vi "initialize.vi"(7 "mode":T1, 8 "log path":path, 9 "pathCtrl":path=path "/Users/philippe/Desktop/LV_Quanser/biquadsff.so", 10 "pathDataCtrl":path=path "/Users/philippe/Desktop/LV_Quanser/biquadsff.so") -> (3 "Qube":refnum<class "Qube.lvclass">)   [LabVIEW 2020, in "Qube.lvclass"]
uses:
  Qube.lvclass
  mode.ctl
  Qube.lvclass/Qube.ctl
  <vilib>/Quanser/Rapid Control Prototyping Toolkit/hardware/HIL Board/HIL Board.lvclass
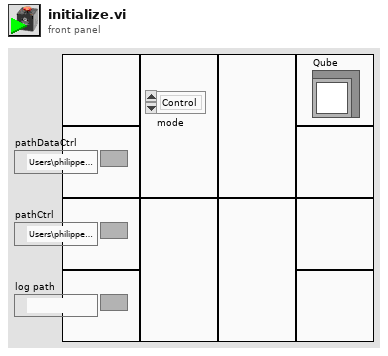
[diagram p1: front panel]
types:
  T1 = typedef "Qube.lvclass/mode.ctl" = enum16{"Control", "Identify"}
  T2 = enum16{"open", "replace", "create", "open or create", "replace or create", "replace or create with confirmation"}
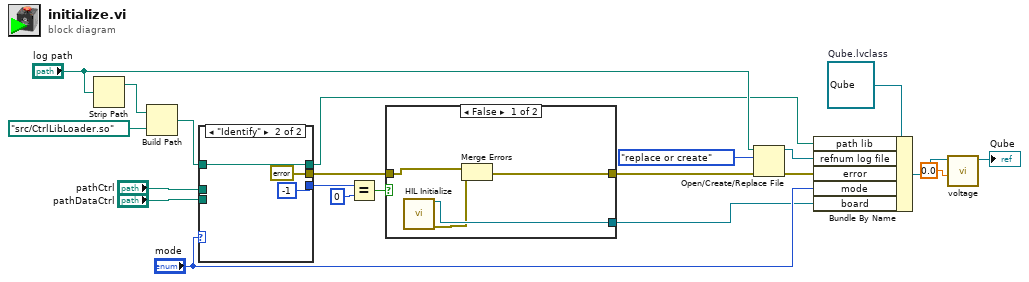
[diagram p0: block diagram]
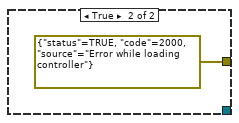
[diagram p2: hidden frame]
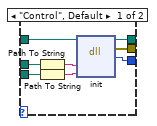
[diagram p3: hidden frame]
diagram:
  w20 = refnum<class "Qube.lvclass"> refnum  # Qube.lvclass
  n1 = Strip Path(path="log path") -> (stripped path=w16:path)  [unwired: 1 out]
  n2 = Build Path(base path=w16, name or relative path=path "src/CtrlLibLoader.so") -> (appended path=w13:path)
  n3 = case shown="\"Identify\"" "mode" {
    tunnel: "pathCtrl" -> [w26 _]
    tunnel: [w23 w31] -> w2
    tunnel: [w24 errorcluster {"status"=FALSE, "code"=0, "source"=""} ("error out")] -> w4
    tunnel: "pathDataCtrl" -> [w27 _]
    tunnel: w13 -> [w25 w31]
    tunnel: [w22 -1 ("return type")] -> w7
    frame "Control", Default {
      n4 = Path To String(path=w26) -> (string=w28:string)
      n5 = Path To String(path=w27) -> (string=w29:string)
      n6 = dll-call lib="Users/philippe/Desktop/cpp/LibLoader/libLoader.so" fn="init"(path in=w25, "pathLib"=w28, "pathInit"=w29) -> (path out=w23:path, error out=w24:errorcluster, "return type"=w22:i32)  [unwired: 4 in]
    }
    frame "Identify" {
    }
  }
  n7 = Equal?(x=w7, y=0) -> (x = y?=w5:bool)
  n8 = case shown="False" w5 {
    tunnel: w4 -> [w34 _]
    tunnel: [w35 errorcluster {"status"=TRUE, "code"=2000, "source"="Error while loading controller"} ("error out")] -> w3
    tunnel: [w36 _] -> w1
    frame False {
      n9 = call "HIL Initialize"() -> ("board out"=w36:refnum<class "HIL Board.lvclass">, "error out"=w33:errorcluster)  [unwired: 14 in]
      n10 = Merge Errors(w34, w33) -> (w35:errorcluster)
    }
    frame True {
    }
  }
  n11 = Open/Create/Replace File(file path (use dialog)="log path", error in=w3, operation (0:open)=T2."replace or create") -> (refnum out=w11:refnum<file>, error out=w10:errorcluster)  [unwired: 3 in, 1 out]
  n12 = Bundle By Name(cluster=w20, "path lib"=w2, "refnum log file"=w11, "error"=w10, "mode"="mode", "board"=w1) -> (w19:refnum<class "Qube.lvclass">)
  n13 = call "voltage.vi"("u"=0.0, "Qube"=w19) -> ("Qube"=→"Qube":refnum<class "Qube.lvclass">)  [unwired: 9 in]
